vi "Average Velocity.vi"() -> (3 "Average Velocity":dbl)   [LabVIEW 2014]
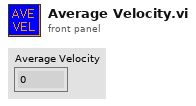
[diagram p1: front panel]
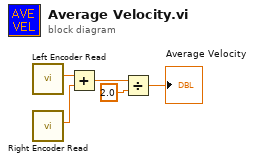
[diagram p0: block diagram]
diagram:
  n1 = call "Left Encoder Read.vi"() -> ("Rate"=w5:dbl)  [unwired: 8 in, 3 out]
  n2 = call "Right Encoder Read.vi"() -> ("Rate"=w4:dbl)  [unwired: 8 in, 3 out]
  n3 = Add(x=w5, y=w4) -> (x+y=w3:dbl)
  n4 = Divide(x=w3, y=2.0) -> (x/y=→"Average Velocity":dbl)
